vi "LQR_with_integrator.vi"() -> ()   [LabVIEW 2021]
uses:
  <vilib>/Simulation/Scripting/Companion Diagram/SimConfigNode/SimParams.ctl
  <vilib>/Simulation/Scripting/Companion Diagram/SimConfigNode/_simSolvers.ctl
  <vilib>/Simulation/Implementation/Shared/SIMSCR Execution Mode.ctl
  <vilib>/Simulation/Param Hierarchy/Typedefs/SIMPH Param Control Actions.ctl
  <vilib>/Simulation/Implementation/Shared/NILVSim_ParamChanged.vi
  <vilib>/Simulation/Implementation/Shared/NILVSIM_BeginStep.vi
  <vilib>/Simulation/DataSources/Implementation/NILVSim Step.llb/SIM Step (scalar).vi
  <vilib>/Simulation/ContinuousLinear/Implementation/NILVSim State Space.llb/SIM State Space Distributor (CD).vi
  <vilib>/Simulation/SignalDisplay/Implementation/NILVSim Time Waveform.llb/SIM Time Waveform (vector).vi
  <vilib>/Simulation/SignalArithmetic/Implementation/NILVSim Gain.llb/SIM Gain (vector,MatrixGain).vi
  <vilib>/Simulation/SignalArithmetic/Implementation/NILVSim Gain.llb/SIM Gain (vector,ScalarGain).vi
  <vilib>/Simulation/ContinuousLinear/Implementation/NILVSim State Space.llb/SIM State Space Collector (CD).vi
  <vilib>/Simulation/Implementation/Shared/NILVSim_Manager.vi
  <vilib>/Utility/error.llb/Clear Errors.vi
  <vilib>/Simulation/Implementation/Shared/NILVSim_FinalizeModel.vi
  <vilib>/addons/Control Design/_Model Construction/Model Creation.llb/Model Creation SubVI/cd_Create State Space Model.vi
  <vilib>/addons/Control Design/_Dynamic Analysis/Dynamic Analysis.llb/Dynamic Analysis subVI/cd_Poles (State-Space).vi
  <vilib>/addons/Control Design/_Dynamic Analysis/Dynamic Analysis.llb/Dynamic Analysis subVI/cd_Pole-Zero Map (State-Space).vi
  <vilib>/addons/Control Design/_Utility/Model Viewer.llb/Model Viewer SubVI/cd_Draw State-Space Equation (SS).vi
  <vilib>/addons/Control Design/_State Feedback Control/State Feedback Control.llb/State Feedback Control SubVis/cd_Linear Quadratic Regulator.vi
  <vilib>/Simulation/Implementation/Shared/SIM Unbundle Sim Info.vi
  <vilib>/Simulation/Implementation/Shared/NILVSim_Initialize.vi
  <vilib>/Simulation/Utility/Implementation/NILVSim Get Time and IsAcceptedStep.vi
  <vilib>/Simulation/Implementation/Shared/SIMSH Read Queue.vi
  <vilib>/Simulation/Implementation/Shared/NILVSim_GetModelError.vi
  <vilib>/Simulation/Implementation/Shared/SIM Bundle Sim Info.vi
  <vilib>/Simulation/Scripting/Companion Diagram/SimConfigNode/SimDog.xnode
  <vilib>/Simulation/Implementation/XNodeFramework/SimXNode/SimX.xnode
  <vilib>/addons/Control Design/_Model Construction/NI_LinSys_Model Creation.lvlib
  <vilib>/addons/Control Design/_State-Space Analysis/NI_CD_State-Space Analysis.lvlib
  <vilib>/addons/Control Design/_Utility/NI_CD_Model Viewer.lvlib
  <vilib>/addons/Control Design/_Dynamic Analysis/NI_CD_Dynamic Analysis.lvlib
  <vilib>/addons/Control Design/_Model Construction/Model Typedefs.llb/CD General Elements.ctl
  <vilib>/addons/Control Design/_Model Construction/NI_LinSys_Model Typedefs.lvlib
  <vilib>/addons/Control Design/_Model Construction/Model Typedefs.llb/CD State Space Model (MIMO).ctl
  <vilib>/Simulation/ContinuousLinear/Implementation/NILVSim State Space.llb/SIM State Space (CD).vi
  <vilib>/addons/Control Design/_State Feedback Control/NI_CD_State Feedback Control.lvlib
  <vilib>/Simulation/Implementation/Shared/NI_SIM_Implementation.lvlib
panel:
  out "open loop Poles":cdb[](array[numeric])=[4.536518488885502+0.0i, -4.536518488885502+0.0i, 0.0+0.0i, 0.0+0.0i] format="%.3f"
  out "control action":waveform(dbl)[](graph)=[{"t0"=timestamp(10 s since 1904-01-01), "dt"=1.0, "Y"=[0.00023247350085175012]}]
  out "Riccati Solution (X)":dbl[][](array[numeric])=[[2.72542242641773, 11.580523530125003, 3.2139637012103544, 2.60698185060518], [11.580523530125003, 300.9099653311846, 28.95483668805577, 66.55426261588948], [3.2139637012103544, 28.95483668805577, 7.577722674468687, 6.514283763652088], [2.60698185060518, 66.55426261588948, 6.514283763652088, 14.837665411951072]] format="%.2f"
  in  "Weighting Type":T1(ring)
  out "states":waveform(dbl)[](graph)=[{"t0"=timestamp(10 s since 1904-01-01), "dt"=1.0, "Y"=[0.10090947704884533]}, {"t0"=timestamp(10 s since 1904-01-01), "dt"=1.0, "Y"=[1.0385159329453754e-05]}, {"t0"=timestamp(10 s since 1904-01-01), "dt"=1.0, "Y"=[-0.0005009091469088976]}, {"t0"=timestamp(10 s since 1904-01-01), "dt"=1.0, "Y"=[1.2724739867584442e-05]}]
  in  "R":dbl[][](array[numeric])=[[1.0]] format="%.2f"
  in  "Q":dbl[][](array[numeric])=[[1.0, 0.0, 0.0, 0.0], [0.0, 1.0, 0.0, 0.0], [0.0, 0.0, 1.0, 0.0], [0.0, 0.0, 0.0, 1.0]] format="%.2f"
  out "output array":dbl[][](array[numeric])=[[0.0, -52.0768442718616, -2.7254224264177447, -11.580523530125028]]
  out "element":dbl=-1.0000000000000027
  in  "refernce":dbl=0.1
  out "Servo System":waveform(dbl)[](graph)=[{"t0"=timestamp(10 s since 1904-01-01), "dt"=1.0, "Y"=[0.10090947704884533]}]
  out "System":cluster{dbl[], dbl[]}[](graph)=[{[4.536518488885502, -4.536518488885502, 0.0, 0.0], [0.0, 0.0, 0.0, 0.0]}, {[-4.42718872423573, 4.427188724235731], [0.0, 0.0]}]
  out "Gain":dbl[][](array[numeric])=[[-1.0000000000000027, -52.0768442718616, -2.7254224264177447, -11.580523530125028]] format="%.2f"
  out "State  Space Model":picture
  out "Transformed Model":picture
  in  "Form Type":u16(ring)=2 items=["Modal"=0, "Companion"=5, "Controllability"=1, "Controller Companion"=2, "Observability"=3, "Observer Companion"=4]
  out "Transformation Matrix (T)":dbl[][](array[numeric])=[[-0.0, -0.0, -0.0, -1.0], [-0.0, -1.0, 0.0, 0.0], [-0.0, -0.0, -0.10204081632653063, -0.051020408163265314], [-0.10204081632653063, -0.051020408163265314, 0.0, 0.0]] format="%.2f"
  out "Is Controllable?":bool=TRUE
  out "Controllability Matrix":dbl[][](array[numeric])=[[0.0, 0.5, 0.0, 0.49], [0.0, -1.0, 0.0, -20.58], [0.5, 0.0, 0.49, 0.0], [-1.0, 0.0, -20.58, 0.0]] format="%.2f"
  in  "D":dbl[][](array[numeric])=[[0.0]] format="%#.5g"
  in  "C":dbl[][](array[numeric])=[[1.0, 0.0, 0.0, 0.0]] format="%#.5g"
  in  "B":dbl[][](array[numeric])=[[0.0], [0.0], [0.5], [-1.0]] format="%#.5g"
  in  "A":dbl[][](array[numeric])=[[0.0, 0.0, 1.0, 0.0], [0.0, 0.0, 0.0, 1.0], [0.0, -0.49, 0.0, 0.0], [0.0, 20.58, 0.0, 0.0]] format="%#.5g"
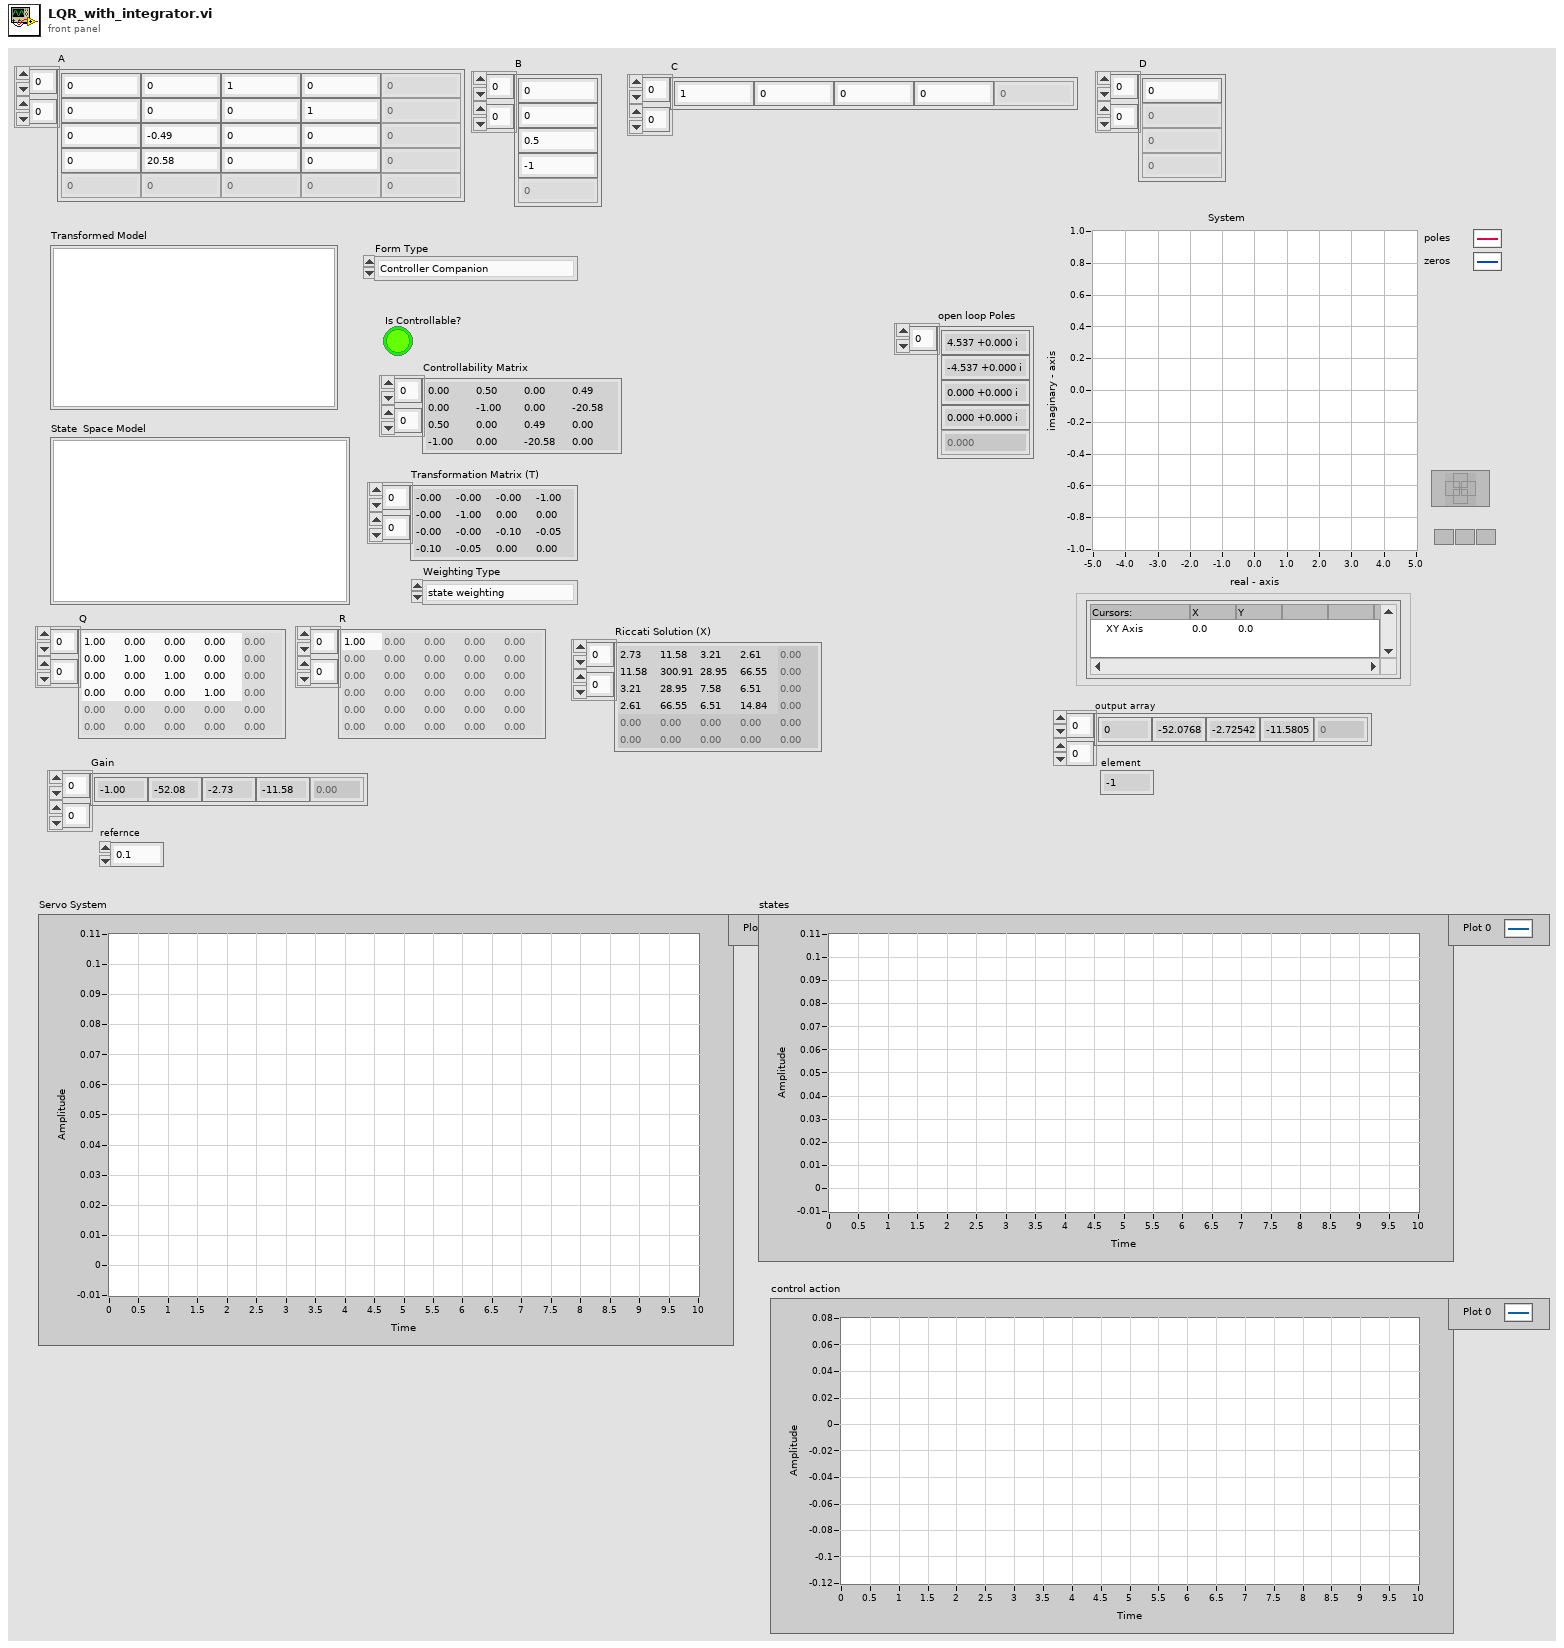
[diagram p1: front panel]
types:
  T1 = enum16{"state weighting", "output weighting, Dim Q = Ny", "output weighting, Dim Q = Nx"}
  T2 = typedef "NI_LinSys_Model Typedefs.lvlib/CD State Space Model (MIMO).ctl" = cluster{"properties":T3, "A":dbl[][], "B":dbl[][], "C":dbl[][], "D":dbl[][], "StateNames":string[], "Transport Delay":dbl[][]}
  T3 = typedef "NI_LinSys_Model Typedefs.lvlib/CD General Elements.ctl" = cluster{"Model name":string, "Input names":string[], "Output names":string[], "Input Delays":dbl[], "Output Delays":dbl[], "Sampling Time":dbl, "Notes":string}
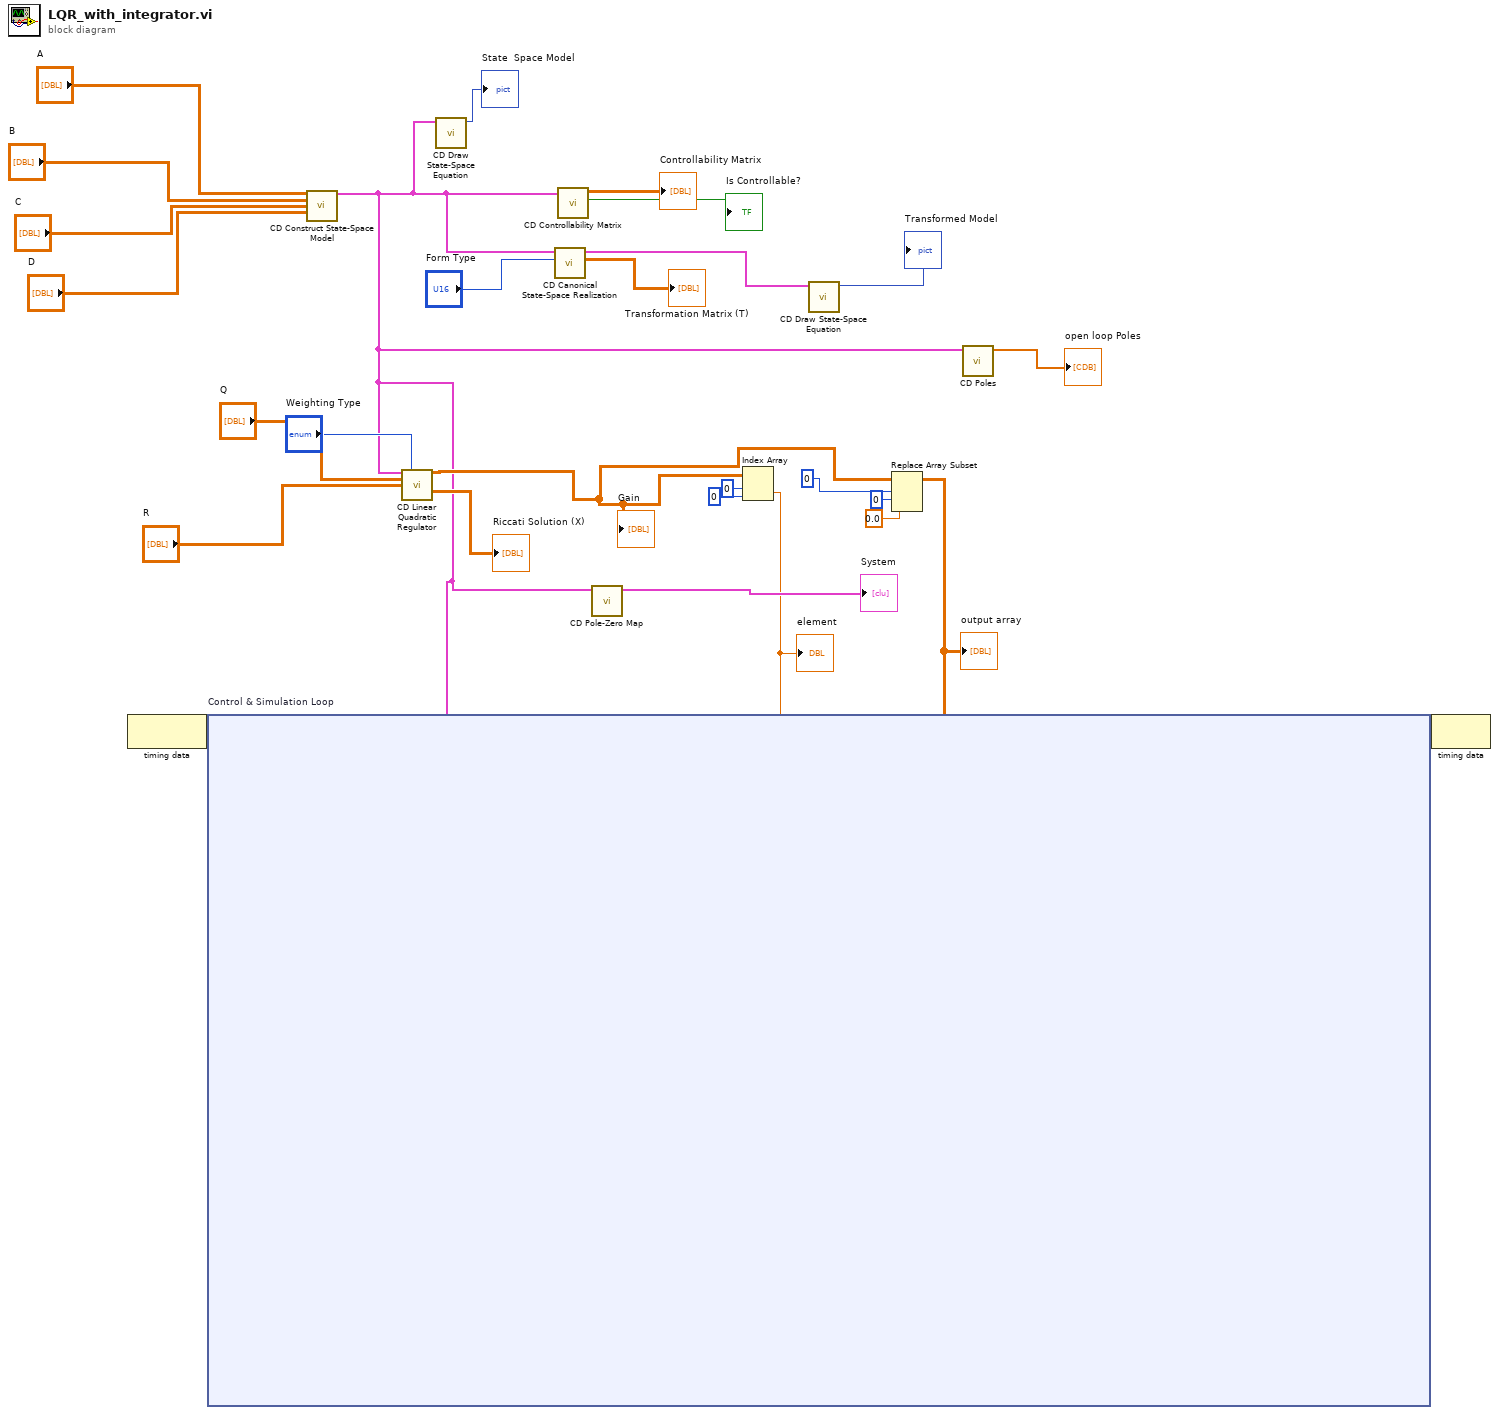
[diagram p0: block diagram]
diagram:
  n1 = node-c288() -> (w16:variant)  [unwired: 1 in]
  n2 = call-poly <vilib>:"CD Construct State-Space Model.vi"("A"="A", "B"="B", "C"="C", "D"="D") -> ("State-Space Model"=w2:T2)  [unwired: 10 in, 1 out]
  n3 = call-poly <vilib>:"CD Linear Quadratic Regulator.vi"("State-Space Model"=w2, "Weighting Type"="Weighting Type", "Q"="Q", "R"="R") -> ("Optimal Gain (K)"=w7:dbl[][], "Riccati Solution (X)"=→"Riccati Solution (X)":dbl[][])  [unwired: 8 in, 2 out]
  "Gain" <- w7
  n4 = call-poly <vilib>:"CD Draw State-Space Equation.vi"("State-Space Model"=w2) -> ("Equation"=→"State  Space Model":picture)  [unwired: 8 in, 2 out]
  n5 = call <vilib>:"CD Canonical State-Space Realization.vi"("Form Type"="Form Type", "State-Space Model"=w2) -> ("Transformation Matrix (T)"=→"Transformation Matrix (T)":dbl[][], "Transformed Model"=w23:T2)  [unwired: 7 in, 1 out]
  n6 = call <vilib>:"CD Controllability Matrix.vi"("State-Space Model"=w2) -> ("Is Controllable?"=→"Is Controllable?":bool, "Controllability Matrix"=→"Controllability Matrix":dbl[][])  [unwired: 7 in, 2 out]
  n7 = call-poly <vilib>:"CD Pole-Zero Map.vi"("State-Space Model"=w2) -> ("Pole-Zero Map"=→"System":cluster{dbl[], dbl[]}[])  [unwired: 7 in, 3 out]
  n8 = Index Array(array=w7, index (row)=0, index (col)=0 ("disabled index (col)")) -> (element=w13:dbl)
  "element" <- w13
  n9 = call-poly <vilib>:"CD Draw State-Space Equation.vi"("State-Space Model"=w23) -> ("Equation"=→"Transformed Model":picture)  [unwired: 8 in, 2 out]
  n10 = Replace Array Subset(array=w7, new element=0.0 ("new element/subarray"), index (row)=0, index (col)=0 ("disabled index (col)")) -> (w11:dbl[][])
  "output array" <- w11
  n11 = node-c254 "Control & Simulation Loop"(w16, w2, w13, w11) -> (w15:variant)
  n12 = call-poly <vilib>:"CD Poles.vi"("State-Space Model"=w2) -> ("Poles"=→"open loop Poles":cdb[])  [unwired: 9 in, 1 out]
  n13 = node-c288(w15) -> ()  [unwired: 1 out]
